vi "Wheel Type String to Ring.vi"(11 "wheel type":string) -> (3 "wheel type_ring":T1 items=["Fixed", "Steering", "Caster", "Mecanum", "Omni", "<Multiple>"])   [LabVIEW 2017, in "NI_Robotics_Configure Steering Frame.lvlib" / "User Defined Frame Subpanel.lvlib"]
uses:
  <vilib>/robotics/Dialog/Configure Steering Frame/User Defined Frame Subpanel/User Defined Frame Subpanel.lvlib
  <vilib>/robotics/Dialog/Configure Steering Frame/Wheel Type.ctl
  <vilib>/robotics/Dialog/Configure Steering Frame/NI_Robotics_Configure Steering Frame.lvlib
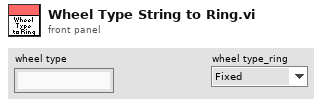
[diagram p1: front panel]
types:
  T1 = typedef "NI_Robotics_Configure Steering Frame.lvlib/Wheel Type.ctl" = u16
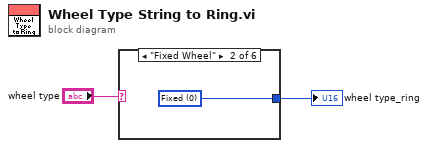
[diagram p0: block diagram]
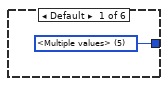
[diagram p2: hidden frame]
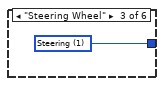
[diagram p3: hidden frame]
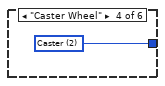
[diagram p4: hidden frame]
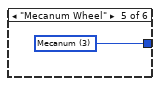
[diagram p5: hidden frame]
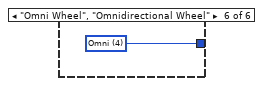
[diagram p6: hidden frame]
diagram:
  n1 = case shown="\"Fixed Wheel\"" "wheel type" {
    tunnel: [w3 w4 w5 w6 w7 w8] -> w1
    frame Default {
      w3 = T1 5 items=["Fixed", "Steering", "Caster", "Mecanum", "Omni", "<Multiple values>"] ("wheel type")
    }
    frame "Fixed Wheel" {
      w4 = T1 0 items=["Fixed", "Steering", "Caster", "Mecanum", "Omni", "<Multiple values>"] ("wheel type")
    }
    frame "Steering Wheel" {
      w5 = T1 1 items=["Fixed", "Steering", "Caster", "Mecanum", "Omni", "<Multiple values>"] ("wheel type")
    }
    frame "Caster Wheel" {
      w6 = T1 2 items=["Fixed", "Steering", "Caster", "Mecanum", "Omni", "<Multiple values>"] ("wheel type")
    }
    frame "Mecanum Wheel" {
      w7 = T1 3 items=["Fixed", "Steering", "Caster", "Mecanum", "Omni", "<Multiple values>"] ("wheel type")
    }
    frame "Omni Wheel", "Omnidirectional Wheel" {
      w8 = T1 4 items=["Fixed", "Steering", "Caster", "Mecanum", "Omni", "<Multiple values>"] ("wheel type")
    }
  }
  "wheel type_ring" <- w1
